vi "Lab Panel V5.24.2.vi"() -> ()   [LabVIEW 2013] (continued)
                          tunnel: w873 -> [_ w886]
                          tunnel: w872 -> [_ w885]
                          tunnel: [errorcluster {"status"=FALSE, "code"=0, "source"=""} ("error out") w884] -> w871
                          tunnel: w870 -> [_ w883]
                          tunnel: w869 -> [_ w882]
                          tunnel: w868 -> [_ w881]
                          tunnel: w867 -> [_ w880]
                          tunnel: w865 -> [_ w879]
                          frame False {
                            w877 = FALSE
                            n583 = local write "RUN LAB01-2"(w877) -> ()
                            n584 = local write "run lab01-2"(w877) -> ()
                          }
                          frame True {
                            n585 = stacked-sequence {
                              seq-local: [w890 _ _ _ _] -> [_ w914 _ _ _]
                              tunnel: w889 -> [w895 _ _ _ _]
                              tunnel: w888 -> [w892 _ _ _ _]
                              tunnel: w887 -> [w905 _ _ _ _]
                              tunnel: w886 -> [w898 _ _ _ _]
                              tunnel: w885 -> [w893 _ _ _ _]
                              tunnel: [_ w909 _ _ _] -> w884
                              tunnel: w883 -> [_ _ _ w936 _]
                              tunnel: w882 -> [_ _ _ w935 _]
                              tunnel: w881 -> [_ _ _ w934 _]
                              tunnel: w880 -> [_ _ _ _ _]
                              tunnel: w879 -> [_ _ _ _ w949]
                              frame #0 {
                                w891 = "\\"
                                n586 = local read "SET LAB01-2"() -> (w900:T5)
                                n587 = case shown="\"CYCLE TEST\"" w905 {
                                tunnel: ["L01-2-CHART TEST-" "L01-2-CYCLE TEST-" "L01-2-T-RISE TEST-"] -> w901
                                frame "CHART TEST", Default {
                                }
                                frame "CYCLE TEST" {
                                }
                                frame "T-RISE TEST" {
                                }
                                }
                                n588 = Unbundle(w900) -> ("DESCRIPTION"=w899:string)  [unwired: 4 out]
                                n589 = Concatenate Strings(w895, "\\", w893, w891, w892, w891) -> (w902:string)
                                n590 = String To Path(string=w902) -> (path=w904:path)
                                n591 = Concatenate Strings(w902, w901, w899, "-", w898, ".tdms") -> (w890:string)
                                n592 = Create Folder(path (use dialog)=w904) -> (error out=w903:errorcluster)  [unwired: 2 in, 2 out]
                                n593 = call <vilib>:"Clear Errors.vi"("error in (no error)"=w903) -> ()  [unwired: 6 in, 1 out]
                                n594 = global write "Global 1.vi" "LAB01-2 FILE"(w890) -> ()
                              }
                              frame #1 {
                                (unwired) FALSE
                                n595 = String To Path(string=w914) -> (path=w910:path)
                                n596 = TDMS Open(6:FALSE, 10:T21."create or replace" ("operation (0:open)"), 11:w910) -> (0:w909:errorcluster, 3:→"TDMS LAB01-2":refnum<k34>)  [unwired: 4 in]
                              }
                              frame #2 {
                                n597 = local read "SET LAB01-2"() -> (w920:T5)
                                n598 = local read "TDMS LAB01-2"() -> (w931:refnum<k34>)
                                n599 = Build Array("Testers Name", "Description", "Set Test Cycles", "T-Rise minutes", "T-Rise Deg C") -> (w921:string[])
                                n600 = Unbundle(w920) -> ("NAME"=w919:string, "DESCRIPTION"=w918:string, "CYCLES"=w917:dbl, "T-RISE mins"=w916:dbl, "T-RISE deg C"=w915:dbl)
                                n601 = Number To Decimal String(number=w917) -> (decimal integer string=w930:string)  [unwired: 1 in]
                                n602 = Number To Decimal String(number=w916) -> (decimal integer string=w929:string)  [unwired: 1 in]
                                n603 = Number To Decimal String(number=w915) -> (decimal integer string=w928:string)  [unwired: 1 in]
                                n604 = Build Array(w919, w918, w930, w929, w928) -> (w927:string[])
                                n605 = TDMS Set Properties(5:w927, 7:w921, 11:w931) -> ()  [unwired: 3 in, 4 out]
                              }
                              frame #3 {
                                n606 = local read "DISP LAB01-2"() -> (w933:T4)
                                n607 = Concatenate Strings("LAB01-2  ", w936) -> (w937:string)
                                n608 = Two Button Dialog(message=w937, 1:w934, 2:w935) -> (T button?=w939:bool)
                                n609 = case shown="True" w939 {
                                tunnel: w933 -> [w946 w947]
                                tunnel: [w946 w947] -> w943
                                tunnel: [w945 w948] -> w942
                                tunnel: [w944 w948] -> w941
                                frame False {
                                n610 = Unbundle(w946) -> ("CYCLE"=w945:dbl, "MINS"=w944:dbl)  [unwired: 1 out]
                                }
                                frame True {
                                w948 = 0.0
                                }
                                }
                                n611 = Bundle(cluster=w943, "CYCLE"=w942, "MINS"=w941, "STATUS"="RUN") -> (w932:T4)
                                n612 = local write "DISP LAB01-2"(w932) -> ()
                              }
                              frame #4 {
                                n613 = local read "TEMP START LAB01-2"() -> (w951:cluster{"TL":dbl, "TN":dbl})
                                n614 = Bundle(cluster=w951, "TL"=w949, "TN"=w949) -> (w950:cluster{"TL":dbl, "TN":dbl})
                                n615 = local write "TEMP START LAB01-2"(w950) -> ()
                              }
                            }
                          }
                        }
                      }
                    }
                  }
                }
              }
              event "RUN LAB02-1": Value Change {
                n616 = event-data() -> ("NewVal"=w957:bool)  [unwired: 1 in, 5 out]
                n617 = local read "SIG LAB02-1"() -> (w953:T2)
                n618 = case shown="True" w957 {
                  tunnel: w963 -> [_ w1001]
                  tunnel: w962 -> [_ w1000]
                  tunnel: w960 -> [w965 w999]
                  tunnel: w961 -> [_ w998]
                  tunnel: w959 -> [_ w997]
                  tunnel: [w964 w996] -> w958
                  tunnel: w956 -> [_ w995]
                  tunnel: w955 -> [_ w994]
                  tunnel: w954 -> [_ w993]
                  tunnel: w953 -> [_ w992]
                  tunnel: w952 -> [_ w991]
                  frame False {
                    # "stop test"
                    n619 = stacked-sequence {
                      tunnel: w965 -> [w974 _]
                      tunnel: [w966 _] -> w964
                      frame #0 {
                        n620 = local read "DISP LAB02-1"() -> (w973:T4)
                        n621 = Unbundle(w973) -> ("CYCLE"=w971:dbl, "MINS"=w972:dbl)  [unwired: 1 out]
                        n622 = case shown="\"CYCLE TEST\"" w974 {
                          tunnel: w972 -> [_ _ w981]
                          tunnel: w971 -> [w979 w980 _]
                          tunnel: [w979 w980 w981] -> w970
                          frame "CHART TEST", Default {
                          }
                          frame "CYCLE TEST" {
                          }
                          frame "T-RISE TEST" {
                          }
                        }
                        n623 = local read "TDMS LAB02-1"() -> (w978:refnum<k34>)
                        n624 = Build Array("STOPPED") -> (w975:string[])
                        n625 = Build Array(w970) -> (w969:dbl[])
                        n626 = TDMS Write(0:w978, 5:"TEST RESULT", 7:w975, 9:w969) -> (4:w967:refnum<k34>, 15:w968:errorcluster)  [unwired: 2 in, 2 out]
                        n627 = TDMS Close(8:w968, 11:w967) -> (0:w966:errorcluster)  [unwired: 1 out]
                      }
                      frame #1 {
                        n628 = local read "DISP LAB02-1"() -> (w985:T4)
                        n629 = stacked-sequence {
                          tunnel: "LAB02-1" -> [w987 w989]
                          frame #0 {
                            n630 = call "sub vi - defrag tdms v1.vi"("panel id"=w987) -> ("error out"=w986:errorcluster)  [unwired: 10 in]
                            n631 = local write "data file error"(w986) -> ()
                          }
                          frame #1 {
                            n632 = local write "RESULT LAB02-1"(FALSE) -> ()
                            n633 = call "Save data file (stop) v3.vi"("panel id"=w989) -> ("network file save error"=w988:errorcluster)  [unwired: 9 in, 1 out]
                            n634 = local write "data file error"(w988) -> ()
                          }
                        }
                        n635 = Bundle(cluster=w985, "STATUS"="STOP") -> (w983:T4)  [unwired: 2 in]
                        n636 = local write "DISP LAB02-1"(w983) -> ()
                      }
                    }
                  }
                  frame True {
                    n637 = stacked-sequence {
                      seq-local: [w1003 _] -> [_ w1007]
                      tunnel: w1001 -> [_ w1017]
                      tunnel: w1000 -> [_ w1016]
                      tunnel: w999 -> [_ w1015]
                      tunnel: w998 -> [_ w1014]
                      tunnel: w997 -> [_ w1013]
                      tunnel: [_ w1012] -> w996
                      tunnel: w995 -> [_ w1011]
                      tunnel: w994 -> [_ w1010]
                      tunnel: w993 -> [_ w1009]
                      tunnel: w992 -> [w1002 w1008]
                      tunnel: w991 -> [_ w1006]
                      frame #0 {
                        n638 = Unbundle(w1002) -> ("AMPS"=w1005:dbl)  [unwired: 4 out]
                        n639 = call "Check For Amps on v1.vi"("ID"="LAB02-1", "amps"=w1005) -> ("amps"=w1003:bool)  [unwired: 9 in]
                      }
                      frame #1 {
                        n640 = case shown="True" w1007 {
                          tunnel: w1017 -> [_ w1030]
                          tunnel: w1016 -> [_ w1029]
                          tunnel: w1015 -> [_ w1028]
                          tunnel: w1014 -> [_ w1027]
                          tunnel: w1013 -> [_ w1026]
                          tunnel: [errorcluster {"status"=FALSE, "code"=0, "source"=""} ("error out") w1025] -> w1012
                          tunnel: w1011 -> [_ w1024]
                          tunnel: w1010 -> [_ w1023]
                          tunnel: w1009 -> [_ w1022]
                          tunnel: w1008 -> [_ w1021]
                          tunnel: w1006 -> [_ w1020]
                          frame False {
                            w1019 = FALSE
                            n641 = local write "RUN LAB02-1"(w1019) -> ()
                            n642 = local write "run lab02-1"(w1019) -> ()
                          }
                          frame True {
                            n643 = stacked-sequence {
                              seq-local: [w1031 _ _ _ _] -> [_ w1055 _ _ _]
                              tunnel: w1030 -> [w1036 _ _ _ _]
                              tunnel: w1029 -> [w1033 _ _ _ _]
                              tunnel: w1028 -> [w1046 _ _ _ _]
                              tunnel: w1027 -> [w1039 _ _ _ _]
                              tunnel: w1026 -> [w1034 _ _ _ _]
                              tunnel: [_ w1050 _ _ _] -> w1025
                              tunnel: w1024 -> [_ _ _ w1076 _]
                              tunnel: w1023 -> [_ _ _ w1075 _]
                              tunnel: w1022 -> [_ _ _ w1074 _]
                              tunnel: w1021 -> [_ _ _ _ _]
                              tunnel: w1020 -> [_ _ _ _ w1090]
                              frame #0 {
                                w1032 = "\\"
                                n644 = local read "SET LAB02-1"() -> (w1041:T5)
                                n645 = case shown="\"CYCLE TEST\"" w1046 {
                                tunnel: ["L02-1-CHART TEST-" "L02-1-CYCLE TEST-" "L02-1-T-RISE TEST-"] -> w1042
                                frame "CHART TEST", Default {
                                }
                                frame "CYCLE TEST" {
                                }
                                frame "T-RISE TEST" {
                                }
                                }
                                n646 = Unbundle(w1041) -> ("DESCRIPTION"=w1040:string)  [unwired: 4 out]
                                n647 = Concatenate Strings(w1036, "\\", w1034, w1032, w1033, w1032) -> (w1043:string)
                                n648 = String To Path(string=w1043) -> (path=w1045:path)
                                n649 = Concatenate Strings(w1043, w1042, w1040, "-", w1039, ".tdms") -> (w1031:string)
                                n650 = Create Folder(path (use dialog)=w1045) -> (error out=w1044:errorcluster)  [unwired: 2 in, 2 out]
                                n651 = global write "Global 1.vi" "LAB02-1 FILE"(w1031) -> ()
                                n652 = call <vilib>:"Clear Errors.vi"("error in (no error)"=w1044) -> ()  [unwired: 6 in, 1 out]
                              }
                              frame #1 {
                                (unwired) FALSE
                                n653 = String To Path(string=w1055) -> (path=w1051:path)
                                n654 = TDMS Open(6:FALSE, 10:T21."create or replace" ("operation (0:open)"), 11:w1051) -> (0:w1050:errorcluster, 3:→"TDMS LAB02-1":refnum<k34>)  [unwired: 4 in]
                              }
                              frame #2 {
                                n655 = local read "SET LAB02-1"() -> (w1061:T5)
                                n656 = local read "TDMS LAB02-1"() -> (w1072:refnum<k34>)
                                n657 = Build Array("Testers Name", "Description", "Set Test Cycles", "T-Rise minutes", "T-Rise Deg C") -> (w1062:string[])
                                n658 = Unbundle(w1061) -> ("NAME"=w1060:string, "DESCRIPTION"=w1059:string, "CYCLES"=w1058:dbl, "T-RISE mins"=w1057:dbl, "T-RISE deg C"=w1056:dbl)
                                n659 = Number To Decimal String(number=w1058) -> (decimal integer string=w1071:string)  [unwired: 1 in]
                                n660 = Number To Decimal String(number=w1057) -> (decimal integer string=w1070:string)  [unwired: 1 in]
                                n661 = Number To Decimal String(number=w1056) -> (decimal integer string=w1069:string)  [unwired: 1 in]
                                n662 = Build Array(w1060, w1059, w1071, w1070, w1069) -> (w1068:string[])
                                n663 = TDMS Set Properties(5:w1068, 7:w1062, 11:w1072) -> ()  [unwired: 3 in, 4 out]
                              }
                              frame #3 {
                                n664 = local read "DISP LAB02-1"() -> (w1077:T4)
                                n665 = Concatenate Strings("LAB02-1  ", w1076) -> (w1078:string)
                                n666 = Two Button Dialog(message=w1078, 1:w1074, 2:w1075) -> (T button?=w1080:bool)
                                n667 = case shown="True" w1080 {
                                tunnel: w1077 -> [w1087 w1088]
                                tunnel: [w1087 w1088] -> w1084
                                tunnel: [w1086 w1089] -> w1083
                                tunnel: [w1085 w1089] -> w1082
                                frame False {
                                n668 = Unbundle(w1087) -> ("CYCLE"=w1086:dbl, "MINS"=w1085:dbl)  [unwired: 1 out]
                                }
                                frame True {
                                w1089 = 0.0
                                }
                                }
                                n669 = Bundle(cluster=w1084, "CYCLE"=w1083, "MINS"=w1082, "STATUS"="RUN") -> (w1073:T4)
                                n670 = local write "DISP LAB02-1"(w1073) -> ()
                              }
                              frame #4 {
                                n671 = local read "TEMP START LAB02-1"() -> (w1092:cluster{"TL":dbl, "TN":dbl})
                                n672 = Bundle(cluster=w1092, "TL"=w1090, "TN"=w1090) -> (w1091:cluster{"TL":dbl, "TN":dbl})
                                n673 = local write "TEMP START LAB02-1"(w1091) -> ()
                              }
                            }
                          }
                        }
                      }
                    }
                  }
                }
                n674 = local write "run lab02-1"(w957) -> ()
              }
              event "RUN LAB02-2": Value Change {
                n675 = event-data() -> ("NewVal"=w1097:bool)  [unwired: 1 in, 5 out]
                n676 = local write "run lab02-2"(w1097) -> ()
                n677 = case shown="True" w1097 {
                  tunnel: w1103 -> [_ w1141]
                  tunnel: w1102 -> [_ w1140]
                  tunnel: w1100 -> [w1105 w1139]
                  tunnel: w1101 -> [_ w1138]
                  tunnel: w1099 -> [_ w1137]
                  tunnel: [w1104 w1136] -> w1098
                  tunnel: w1096 -> [_ w1135]
                  tunnel: w1095 -> [_ w1134]
                  tunnel: w1094 -> [_ w1133]
                  tunnel: w1093 -> [_ w1131]
                  frame False {
                    # "stop test"
                    n678 = stacked-sequence {
                      tunnel: w1105 -> [w1114 _]
                      tunnel: [w1106 _] -> w1104
                      frame #0 {
                        n679 = local read "DISP LAB02-2"() -> (w1113:T4)
                        n680 = Unbundle(w1113) -> ("CYCLE"=w1111:dbl, "MINS"=w1112:dbl)  [unwired: 1 out]
                        n681 = case shown="\"CYCLE TEST\"" w1114 {
                          tunnel: w1112 -> [_ _ w1121]
                          tunnel: w1111 -> [w1119 w1120 _]
                          tunnel: [w1119 w1120 w1121] -> w1110
                          frame "CHART TEST", Default {
                          }
                          frame "CYCLE TEST" {
                          }
                          frame "T-RISE TEST" {
                          }
                        }
                        n682 = local read "TDMS LAB02-2"() -> (w1118:refnum<k34>)
                        n683 = Build Array("STOPPED") -> (w1115:string[])
                        n684 = Build Array(w1110) -> (w1109:dbl[])
                        n685 = TDMS Write(0:w1118, 5:"TEST RESULT", 7:w1115, 9:w1109) -> (4:w1107:refnum<k34>, 15:w1108:errorcluster)  [unwired: 2 in, 2 out]
                        n686 = TDMS Close(8:w1108, 11:w1107) -> (0:w1106:errorcluster)  [unwired: 1 out]
                      }
                      frame #1 {
                        n687 = local read "DISP LAB02-2"() -> (w1125:T4)
                        n688 = stacked-sequence {
                          tunnel: "LAB02-2" -> [w1127 w1129]
                          frame #0 {
                            n689 = call "sub vi - defrag tdms v1.vi"("panel id"=w1127) -> ("error out"=w1126:errorcluster)  [unwired: 10 in]
                            n690 = local write "data file error"(w1126) -> ()
                          }
                          frame #1 {
                            n691 = call "Save data file (stop) v3.vi"("panel id"=w1129) -> ("network file save error"=w1128:errorcluster)  [unwired: 9 in, 1 out]
                            n692 = local write "RESULT LAB02-2"(FALSE) -> ()
                            n693 = local write "data file error"(w1128) -> ()
                          }
                        }
                        n694 = Bundle(cluster=w1125, "STATUS"="STOP") -> (w1123:T4)  [unwired: 2 in]
                        n695 = local write "DISP LAB02-2"(w1123) -> ()
                      }
                    }
                  }
                  frame True {
                    n696 = local read "SIG LAB02-2"() -> (w1132:T2)
                    n697 = stacked-sequence {
                      seq-local: [w1143 _] -> [_ w1147]
                      tunnel: w1141 -> [_ w1157]
                      tunnel: w1140 -> [_ w1156]
                      tunnel: w1139 -> [_ w1155]
                      tunnel: w1138 -> [_ w1154]
                      tunnel: w1137 -> [_ w1153]
                      tunnel: [_ w1152] -> w1136
                      tunnel: w1135 -> [_ w1151]
                      tunnel: w1134 -> [_ w1150]
                      tunnel: w1133 -> [_ w1149]
                      tunnel: w1132 -> [w1142 w1148]
                      tunnel: w1131 -> [_ w1146]
                      frame #0 {
                        n698 = Unbundle(w1142) -> ("AMPS"=w1145:dbl)  [unwired: 4 out]
                        n699 = call "Check For Amps on v1.vi"("ID"="LAB02-2", "amps"=w1145) -> ("amps"=w1143:bool)  [unwired: 9 in]
                      }
                      frame #1 {
                        n700 = case shown="True" w1147 {
                          tunnel: w1157 -> [_ w1170]
                          tunnel: w1156 -> [_ w1169]
                          tunnel: w1155 -> [_ w1168]
                          tunnel: w1154 -> [_ w1167]
                          tunnel: w1153 -> [_ w1166]
                          tunnel: [errorcluster {"status"=FALSE, "code"=0, "source"=""} ("error out") w1165] -> w1152
                          tunnel: w1151 -> [_ w1164]
                          tunnel: w1150 -> [_ w1163]
                          tunnel: w1149 -> [_ w1162]
                          tunnel: w1148 -> [_ w1161]
                          tunnel: w1146 -> [_ w1160]
                          frame False {
                            w1158 = FALSE
                            n701 = local write "RUN LAB02-2"(w1158) -> ()
                            n702 = local write "run lab02-2"(w1158) -> ()
                          }
                          frame True {
                            n703 = stacked-sequence {
                              seq-local: [w1171 _ _ _ _] -> [_ w1195 _ _ _]
                              tunnel: w1170 -> [w1176 _ _ _ _]
                              tunnel: w1169 -> [w1173 _ _ _ _]
                              tunnel: w1168 -> [w1186 _ _ _ _]
                              tunnel: w1167 -> [w1179 _ _ _ _]
                              tunnel: w1166 -> [w1174 _ _ _ _]
                              tunnel: [_ w1190 _ _ _] -> w1165
                              tunnel: w1164 -> [_ _ _ w1216 _]
                              tunnel: w1163 -> [_ _ _ w1215 _]
                              tunnel: w1162 -> [_ _ _ w1214 _]
                              tunnel: w1161 -> [_ _ _ _ _]
                              tunnel: w1160 -> [_ _ _ _ w1230]
                              frame #0 {
                                w1172 = "\\"
                                n704 = local read "SET LAB02-2"() -> (w1181:T5)
                                n705 = case shown="\"CYCLE TEST\"" w1186 {
                                tunnel: ["L02-2-CHART TEST-" "L02-2-CYCLE TEST-" "L02-2-T-RISE TEST-"] -> w1182
                                frame "CHART TEST", Default {
                                }
                                frame "CYCLE TEST" {
                                }
                                frame "T-RISE TEST" {
                                }
                                }
                                n706 = Unbundle(w1181) -> ("DESCRIPTION"=w1180:string)  [unwired: 4 out]
                                n707 = Concatenate Strings(w1176, "\\", w1174, w1172, w1173, w1172) -> (w1183:string)
                                n708 = String To Path(string=w1183) -> (path=w1185:path)
                                n709 = Concatenate Strings(w1183, w1182, w1180, "-", w1179, ".tdms") -> (w1171:string)
                                n710 = Create Folder(path (use dialog)=w1185) -> (error out=w1184:errorcluster)  [unwired: 2 in, 2 out]
                                n711 = global write "Global 1.vi" "LAB02-2 FILE"(w1171) -> ()
                                n712 = call <vilib>:"Clear Errors.vi"("error in (no error)"=w1184) -> ()  [unwired: 6 in, 1 out]
                              }
                              frame #1 {
                                (unwired) FALSE
                                n713 = String To Path(string=w1195) -> (path=w1191:path)
                                n714 = TDMS Open(6:FALSE, 10:T21."create or replace" ("operation (0:open)"), 11:w1191) -> (0:w1190:errorcluster, 3:→"TDMS LAB02-2":refnum<k34>)  [unwired: 4 in]
                              }
                              frame #2 {
                                n715 = local read "SET LAB02-2"() -> (w1201:T5)
                                n716 = local read "TDMS LAB02-2"() -> (w1212:refnum<k34>)
                                n717 = Build Array("Testers Name", "Description", "Set Test Cycles", "T-Rise minutes", "T-Rise Deg C") -> (w1202:string[])
                                n718 = Unbundle(w1201) -> ("NAME"=w1200:string, "DESCRIPTION"=w1199:string, "CYCLES"=w1198:dbl, "T-RISE mins"=w1197:dbl, "T-RISE deg C"=w1196:dbl)
                                n719 = Number To Decimal String(number=w1198) -> (decimal integer string=w1211:string)  [unwired: 1 in]
                                n720 = Number To Decimal String(number=w1197) -> (decimal integer string=w1210:string)  [unwired: 1 in]
                                n721 = Number To Decimal String(number=w1196) -> (decimal integer string=w1209:string)  [unwired: 1 in]
                                n722 = Build Array(w1200, w1199, w1211, w1210, w1209) -> (w1208:string[])
                                n723 = TDMS Set Properties(5:w1208, 7:w1202, 11:w1212) -> ()  [unwired: 3 in, 4 out]
                              }
                              frame #3 {
                                n724 = local read "DISP LAB02-2"() -> (w1217:T4)
                                n725 = Concatenate Strings("LAB02-2  ", w1216) -> (w1218:string)
                                n726 = Two Button Dialog(message=w1218, 1:w1214, 2:w1215) -> (T button?=w1220:bool)
                                n727 = case shown="True" w1220 {
                                tunnel: w1217 -> [w1227 w1228]
                                tunnel: [w1227 w1228] -> w1224
                                tunnel: [w1226 w1229] -> w1223
                                tunnel: [w1225 w1229] -> w1222
                                frame False {
                                n728 = Unbundle(w1227) -> ("CYCLE"=w1226:dbl, "MINS"=w1225:dbl)  [unwired: 1 out]
                                }
                                frame True {
                                w1229 = 0.0
                                }
                                }
                                n729 = Bundle(cluster=w1224, "CYCLE"=w1223, "MINS"=w1222, "STATUS"="RUN") -> (w1213:T4)
                                n730 = local write "DISP LAB02-2"(w1213) -> ()
                              }
                              frame #4 {
                                n731 = local read "TEMP START LAB02-2"() -> (w1232:cluster{"TL":dbl, "TN":dbl})
                                n732 = Bundle(cluster=w1232, "TL"=w1230, "TN"=w1230) -> (w1231:cluster{"TL":dbl, "TN":dbl})
                                n733 = local write "TEMP START LAB02-2"(w1231) -> ()
                              }
                            }
                          }
                        }
                      }
                    }
                  }
                }
              }
              event "RUN LAB03-1": Value Change {
                n734 = event-data() -> ("NewVal"=w1237:bool)  [unwired: 1 in, 5 out]
                n735 = local write "run lab03-1"(w1237) -> ()
                n736 = case shown="True" w1237 {
                  tunnel: w1243 -> [_ w1281]
                  tunnel: w1242 -> [_ w1280]
                  tunnel: w1240 -> [w1245 w1279]
                  tunnel: w1241 -> [_ w1278]
                  tunnel: w1239 -> [_ w1277]
                  tunnel: [w1244 w1276] -> w1238
                  tunnel: w1236 -> [_ w1275]
                  tunnel: w1235 -> [_ w1274]
                  tunnel: w1234 -> [_ w1273]
                  tunnel: w1233 -> [_ w1271]
                  frame False {
                    # "stop test"
                    n737 = stacked-sequence {
                      tunnel: w1245 -> [w1254 _]
                      tunnel: [w1246 _] -> w1244
                      frame #0 {
                        n738 = local read "DISP LAB03-1"() -> (w1253:T4)
                        n739 = Unbundle(w1253) -> ("CYCLE"=w1251:dbl, "MINS"=w1252:dbl)  [unwired: 1 out]
                        n740 = case shown="\"CYCLE TEST\"" w1254 {
                          tunnel: w1252 -> [_ _ w1261]
                          tunnel: w1251 -> [w1259 w1260 _]
                          tunnel: [w1259 w1260 w1261] -> w1250
                          frame "CHART TEST", Default {
                          }
                          frame "CYCLE TEST" {
                          }
                          frame "T-RISE TEST" {
                          }
                        }
                        n741 = local read "TDMS LAB03-1"() -> (w1258:refnum<k34>)
                        n742 = Build Array("STOPPED") -> (w1255:string[])
                        n743 = Build Array(w1250) -> (w1249:dbl[])
                        n744 = TDMS Write(0:w1258, 5:"TEST RESULT", 7:w1255, 9:w1249) -> (4:w1247:refnum<k34>, 15:w1248:errorcluster)  [unwired: 2 in, 2 out]
                        n745 = TDMS Close(8:w1248, 11:w1247) -> (0:w1246:errorcluster)  [unwired: 1 out]
                      }
                      frame #1 {
                        n746 = local read "DISP LAB03-1"() -> (w1265:T4)
                        n747 = stacked-sequence {
                          tunnel: "LAB03-1" -> [w1267 w1269]
                          frame #0 {
                            n748 = call "sub vi - defrag tdms v1.vi"("panel id"=w1267) -> ("error out"=w1266:errorcluster)  [unwired: 10 in]
                            n749 = local write "data file error"(w1266) -> ()
                          }
                          frame #1 {
                            n750 = call "Save data file (stop) v3.vi"("panel id"=w1269) -> ("network file save error"=w1268:errorcluster)  [unwired: 9 in, 1 out]
                            n751 = local write "RESULT LAB03-1"(FALSE) -> ()
                            n752 = local write "data file error"(w1268) -> ()
                          }
                        }
                        n753 = Bundle(cluster=w1265, "STATUS"="STOP") -> (w1263:T4)  [unwired: 2 in]
                        n754 = local write "DISP LAB03-1"(w1263) -> ()
                      }
                    }
                  }
                  frame True {
                    n755 = local read "SIG LAB03-1"() -> (w1272:T2)
                    n756 = stacked-sequence {
                      seq-local: [w1283 _] -> [_ w1287]
                      tunnel: w1281 -> [_ w1297]
                      tunnel: w1280 -> [_ w1296]
                      tunnel: w1279 -> [_ w1295]
                      tunnel: w1278 -> [_ w1294]
                      tunnel: w1277 -> [_ w1293]
                      tunnel: [_ w1292] -> w1276
                      tunnel: w1275 -> [_ w1291]
                      tunnel: w1274 -> [_ w1290]
                      tunnel: w1273 -> [_ w1289]
                      tunnel: w1272 -> [w1282 w1288]
                      tunnel: w1271 -> [_ w1286]
                      frame #0 {
                        n757 = Unbundle(w1282) -> ("AMPS"=w1285:dbl)  [unwired: 4 out]
                        n758 = call "Check For Amps on v1.vi"("ID"="LAB03-1", "amps"=w1285) -> ("amps"=w1283:bool)  [unwired: 9 in]
                      }
                      frame #1 {
                        n759 = case shown="True" w1287 {
                          tunnel: w1297 -> [_ w1310]
                          tunnel: w1296 -> [_ w1309]
                          tunnel: w1295 -> [_ w1308]
                          tunnel: w1294 -> [_ w1307]
                          tunnel: w1293 -> [_ w1306]
                          tunnel: [errorcluster {"status"=FALSE, "code"=0, "source"=""} ("error out") w1305] -> w1292
                          tunnel: w1291 -> [_ w1304]
                          tunnel: w1290 -> [_ w1303]
                          tunnel: w1289 -> [_ w1302]
                          tunnel: w1288 -> [_ w1301]
                          tunnel: w1286 -> [_ w1300]
                          frame False {
                            w1298 = FALSE
                            n760 = local write "RUN LAB03-1"(w1298) -> ()
                            n761 = local write "run lab03-1"(w1298) -> ()
                          }
                          frame True {
                            n762 = stacked-sequence {
                              seq-local: [w1311 _ _ _ _] -> [_ w1335 _ _ _]
                              tunnel: w1310 -> [w1316 _ _ _ _]
                              tunnel: w1309 -> [w1313 _ _ _ _]
                              tunnel: w1308 -> [w1326 _ _ _ _]
                              tunnel: w1307 -> [w1319 _ _ _ _]
                              tunnel: w1306 -> [w1314 _ _ _ _]
                              tunnel: [_ w1330 _ _ _] -> w1305
                              tunnel: w1304 -> [_ _ _ w1355 _]
                              tunnel: w1303 -> [_ _ _ w1354 _]
                              tunnel: w1302 -> [_ _ _ w1353 _]
                              tunnel: w1301 -> [_ _ _ _ _]
                              tunnel: w1300 -> [_ _ _ _ w1370]
                              frame #0 {
                                w1312 = "\\"
                                n763 = local read "SET LAB03-1"() -> (w1321:T5)
                                n764 = case shown="\"T-RISE TEST\"" w1326 {
                                tunnel: ["L03-1-CHART TEST-" "L03-1-CYCLE TEST-" "L03-1-T-RISE TEST-"] -> w1322
                                frame "CHART TEST", Default {
                                }
                                frame "CYCLE TEST" {
                                }
                                frame "T-RISE TEST" {
                                }
                                }
                                n765 = Unbundle(w1321) -> ("DESCRIPTION"=w1320:string)  [unwired: 4 out]
                                n766 = Concatenate Strings(w1316, "\\", w1314, w1312, w1313, w1312) -> (w1323:string)
                                n767 = String To Path(string=w1323) -> (path=w1325:path)
                                n768 = Concatenate Strings(w1323, w1322, w1320, "-", w1319, ".tdms") -> (w1311:string)
                                n769 = Create Folder(path (use dialog)=w1325) -> (error out=w1324:errorcluster)  [unwired: 2 in, 2 out]
                                n770 = global write "Global 1.vi" "LAB03-1 FILE"(w1311) -> ()
                                n771 = call <vilib>:"Clear Errors.vi"("error in (no error)"=w1324) -> ()  [unwired: 6 in, 1 out]
                              }
                              frame #1 {
                                (unwired) FALSE
                                n772 = String To Path(string=w1335) -> (path=w1331:path)
                                n773 = TDMS Open(6:FALSE, 10:T21."create or replace" ("operation (0:open)"), 11:w1331) -> (0:w1330:errorcluster, 3:→"TDMS LAB03-1":refnum<k34>)  [unwired: 4 in]
                              }
                              frame #2 {
                                n774 = local read "SET LAB03-1"() -> (w1341:T5)
                                n775 = local read "TDMS LAB03-1"() -> (w1352:refnum<k34>)
                                n776 = Build Array("Testers Name", "Description", "Set Test Cycles", "T-Rise minutes", "T-Rise Deg C") -> (w1342:string[])
                                n777 = Unbundle(w1341) -> ("NAME"=w1340:string, "DESCRIPTION"=w1339:string, "CYCLES"=w1338:dbl, "T-RISE mins"=w1337:dbl, "T-RISE deg C"=w1336:dbl)
                                n778 = Number To Decimal String(number=w1338) -> (decimal integer string=w1351:string)  [unwired: 1 in]
                                n779 = Number To Decimal String(number=w1337) -> (decimal integer string=w1350:string)  [unwired: 1 in]
                                n780 = Number To Decimal String(number=w1336) -> (decimal integer string=w1349:string)  [unwired: 1 in]
                                n781 = Build Array(w1340, w1339, w1351, w1350, w1349) -> (w1348:string[])
                                n782 = TDMS Set Properties(5:w1348, 7:w1342, 11:w1352) -> ()  [unwired: 3 in, 4 out]
                              }
                              frame #3 {
                                n783 = local read "DISP LAB03-1"() -> (w1357:T4)
                                n784 = Concatenate Strings("LAB03-1  ", w1355) -> (w1358:string)
                                n785 = Two Button Dialog(message=w1358, 1:w1353, 2:w1354) -> (T button?=w1360:bool)
                                n786 = case shown="True" w1360 {
                                tunnel: w1357 -> [w1367 w1368]
                                tunnel: [w1367 w1368] -> w1364
                                tunnel: [w1366 w1369] -> w1363
                                tunnel: [w1365 w1369] -> w1362
                                frame False {
                                n787 = Unbundle(w1367) -> ("CYCLE"=w1366:dbl, "MINS"=w1365:dbl)  [unwired: 1 out]
                                }
                                frame True {
                                w1369 = 0.0
                                }
                                }
                                n788 = Bundle(cluster=w1364, "CYCLE"=w1363, "MINS"=w1362, "STATUS"="RUN") -> (w1356:T4)
                                n789 = local write "DISP LAB03-1"(w1356) -> ()
                              }
                              frame #4 {
                                n790 = local read "TEMP START LAB03-1"() -> (w1372:cluster{"TL":dbl, "TN":dbl})
                                n791 = Bundle(cluster=w1372, "TL"=w1370, "TN"=w1370) -> (w1371:cluster{"TL":dbl, "TN":dbl})
                                n792 = local write "TEMP START LAB03-1"(w1371) -> ()
                              }
                            }
                          }
                        }
                      }
                    }
                  }
                }
              }
              event "RUN LAB03-2": Value Change {
                n793 = event-data() -> ("NewVal"=w1377:bool)  [unwired: 1 in, 5 out]
                n794 = local write "run lab03-2"(w1377) -> ()
                n795 = case shown="True" w1377 {
                  tunnel: w1383 -> [_ w1421]
                  tunnel: w1382 -> [_ w1420]
                  tunnel: w1380 -> [w1385 w1419]
                  tunnel: w1381 -> [_ w1418]
                  tunnel: w1379 -> [_ w1417]
                  tunnel: [w1384 w1416] -> w1378
                  tunnel: w1376 -> [_ w1415]
                  tunnel: w1375 -> [_ w1414]
                  tunnel: w1374 -> [_ w1413]
                  tunnel: w1373 -> [_ w1411]
                  frame False {
                    # "stop test"
                    n796 = stacked-sequence {
                      tunnel: w1385 -> [w1394 _]
                      tunnel: [w1386 _] -> w1384
                      frame #0 {
                        n797 = local read "DISP LAB03-2"() -> (w1393:T4)
                        n798 = Unbundle(w1393) -> ("CYCLE"=w1391:dbl, "MINS"=w1392:dbl)  [unwired: 1 out]
                        n799 = case shown="\"CYCLE TEST\"" w1394 {
                          tunnel: w1392 -> [_ _ w1401]
                          tunnel: w1391 -> [w1399 w1400 _]
                          tunnel: [w1399 w1400 w1401] -> w1390
                          frame "CHART TEST", Default {
                          }
                          frame "CYCLE TEST" {
                          }
                          frame "T-RISE TEST" {
                          }
                        }
                        n800 = local read "TDMS LAB03-2"() -> (w1398:refnum<k34>)
                        n801 = Build Array("STOPPED") -> (w1395:string[])
                        n802 = Build Array(w1390) -> (w1389:dbl[])
                        n803 = TDMS Write(0:w1398, 5:"TEST RESULT", 7:w1395, 9:w1389) -> (4:w1387:refnum<k34>, 15:w1388:errorcluster)  [unwired: 2 in, 2 out]
                        n804 = TDMS Close(8:w1388, 11:w1387) -> (0:w1386:errorcluster)  [unwired: 1 out]
                      }
                      frame #1 {
                        n805 = local read "DISP LAB03-2"() -> (w1405:T4)
                        n806 = stacked-sequence {
                          tunnel: "LAB03-2" -> [w1407 w1409]
                          frame #0 {
                            n807 = call "sub vi - defrag tdms v1.vi"("panel id"=w1407) -> ("error out"=w1406:errorcluster)  [unwired: 10 in]
                            n808 = local write "data file error"(w1406) -> ()
                          }
                          frame #1 {
                            n809 = call "Save data file (stop) v3.vi"("panel id"=w1409) -> ("network file save error"=w1408:errorcluster)  [unwired: 9 in, 1 out]
                            n810 = local write "RESULT LAB03-2"(FALSE) -> ()
                            n811 = local write "data file error"(w1408) -> ()
                          }
                        }
                        n812 = Bundle(cluster=w1405, "STATUS"="STOP") -> (w1403:T4)  [unwired: 2 in]
                        n813 = local write "DISP LAB03-2"(w1403) -> ()
                      }
                    }
                  }
                  frame True {
                    n814 = local read "SIG LAB03-2"() -> (w1412:T2)
                    n815 = stacked-sequence {
                      seq-local: [w1423 _] -> [_ w1427]
                      tunnel: w1421 -> [_ w1437]
                      tunnel: w1420 -> [_ w1436]
                      tunnel: w1419 -> [_ w1435]
                      tunnel: w1418 -> [_ w1434]
                      tunnel: w1417 -> [_ w1433]
                      tunnel: [_ w1432] -> w1416
                      tunnel: w1415 -> [_ w1431]
                      tunnel: w1414 -> [_ w1430]
                      tunnel: w1413 -> [_ w1429]
                      tunnel: w1412 -> [w1422 w1428]
                      tunnel: w1411 -> [_ w1426]
                      frame #0 {
                        n816 = Unbundle(w1422) -> ("AMPS"=w1425:dbl)  [unwired: 4 out]
                        n817 = call "Check For Amps on v1.vi"("ID"="LAB03-2", "amps"=w1425) -> ("amps"=w1423:bool)  [unwired: 9 in]
                      }
                      frame #1 {
                        n818 = case shown="True" w1427 {
                          tunnel: w1437 -> [_ w1450]
                          tunnel: w1436 -> [_ w1449]
                          tunnel: w1435 -> [_ w1448]
                          tunnel: w1434 -> [_ w1447]
                          tunnel: w1433 -> [_ w1446]
                          tunnel: [errorcluster {"status"=FALSE, "code"=0, "source"=""} ("error out") w1445] -> w1432
                          tunnel: w1431 -> [_ w1444]
                          tunnel: w1430 -> [_ w1443]
                          tunnel: w1429 -> [_ w1442]
                          tunnel: w1428 -> [_ w1441]
                          tunnel: w1426 -> [_ w1440]
                          frame False {
                            w1438 = FALSE
                            n819 = local write "RUN LAB03-2"(w1438) -> ()
                            n820 = local write "run lab03-2"(w1438) -> ()
                          }
                          frame True {
                            n821 = stacked-sequence {
                              seq-local: [w1451 _ _ _ _] -> [_ w1475 _ _ _]
                              tunnel: w1450 -> [w1456 _ _ _ _]
                              tunnel: w1449 -> [w1453 _ _ _ _]
                              tunnel: w1448 -> [w1466 _ _ _ _]
                              tunnel: w1447 -> [w1459 _ _ _ _]
                              tunnel: w1446 -> [w1454 _ _ _ _]
                              tunnel: [_ w1470 _ _ _] -> w1445
                              tunnel: w1444 -> [_ _ _ w1496 _]
                              tunnel: w1443 -> [_ _ _ w1495 _]
                              tunnel: w1442 -> [_ _ _ w1494 _]
                              tunnel: w1441 -> [_ _ _ _ _]
                              tunnel: w1440 -> [_ _ _ _ w1510]
                              frame #0 {
                                w1452 = "\\"
                                n822 = local read "SET LAB03-2"() -> (w1461:T5)
                                n823 = case shown="\"T-RISE TEST\"" w1466 {
                                tunnel: ["L03-2-CHART TEST-" "L03-2-CYCLE TEST-" "L03-2-T-RISE TEST-"] -> w1462
                                frame "CHART TEST", Default {
                                }
                                frame "CYCLE TEST" {
                                }
                                frame "T-RISE TEST" {
                                }
                                }
                                n824 = Unbundle(w1461) -> ("DESCRIPTION"=w1460:string)  [unwired: 4 out]
                                n825 = Concatenate Strings(w1456, "\\", w1454, w1452, w1453, w1452) -> (w1463:string)
                                n826 = String To Path(string=w1463) -> (path=w1465:path)
                                n827 = Concatenate Strings(w1463, w1462, w1460, "-", w1459, ".tdms") -> (w1451:string)
                                n828 = Create Folder(path (use dialog)=w1465) -> (error out=w1464:errorcluster)  [unwired: 2 in, 2 out]
                                n829 = global write "Global 1.vi" "LAB03-2 FILE"(w1451) -> ()
                                n830 = call <vilib>:"Clear Errors.vi"("error in (no error)"=w1464) -> ()  [unwired: 6 in, 1 out]
                              }
                              frame #1 {
                                (unwired) FALSE
                                n831 = String To Path(string=w1475) -> (path=w1471:path)
                                n832 = TDMS Open(6:FALSE, 10:T21."create or replace" ("operation (0:open)"), 11:w1471) -> (0:w1470:errorcluster, 3:→"TDMS LAB03-2":refnum<k34>)  [unwired: 4 in]
                              }
                              frame #2 {
                                n833 = local read "SET LAB03-2"() -> (w1481:T5)
                                n834 = local read "TDMS LAB03-2"() -> (w1492:refnum<k34>)
                                n835 = Build Array("Testers Name", "Description", "Set Test Cycles", "T-Rise minutes", "T-Rise Deg C") -> (w1482:string[])
                                n836 = Unbundle(w1481) -> ("NAME"=w1480:string, "DESCRIPTION"=w1479:string, "CYCLES"=w1478:dbl, "T-RISE mins"=w1477:dbl, "T-RISE deg C"=w1476:dbl)
                                n837 = Number To Decimal String(number=w1478) -> (decimal integer string=w1491:string)  [unwired: 1 in]
                                n838 = Number To Decimal String(number=w1477) -> (decimal integer string=w1490:string)  [unwired: 1 in]
                                n839 = Number To Decimal String(number=w1476) -> (decimal integer string=w1489:string)  [unwired: 1 in]
                                n840 = Build Array(w1480, w1479, w1491, w1490, w1489) -> (w1488:string[])
                                n841 = TDMS Set Properties(5:w1488, 7:w1482, 11:w1492) -> ()  [unwired: 3 in, 4 out]
                              }
                              frame #3 {
                                n842 = local read "DISP LAB03-2"() -> (w1497:T4)
                                n843 = Concatenate Strings("LAB03-2  ", w1496) -> (w1498:string)
                                n844 = Two Button Dialog(message=w1498, 1:w1494, 2:w1495) -> (T button?=w1500:bool)
                                n845 = case shown="True" w1500 {
                                tunnel: w1497 -> [w1507 w1508]
                                tunnel: [w1507 w1508] -> w1504
                                tunnel: [w1506 w1509] -> w1503
                                tunnel: [w1505 w1509] -> w1502
                                frame False {
                                n846 = Unbundle(w1507) -> ("CYCLE"=w1506:dbl, "MINS"=w1505:dbl)  [unwired: 1 out]
                                }
                                frame True {
                                w1509 = 0.0
                                }
                                }
                                n847 = Bundle(cluster=w1504, "CYCLE"=w1503, "MINS"=w1502, "STATUS"="RUN") -> (w1493:T4)
                                n848 = local write "DISP LAB03-2"(w1493) -> ()
                              }
                              frame #4 {
                                n849 = local read "TEMP START LAB03-2"() -> (w1512:cluster{"TL":dbl, "TN":dbl})
                                n850 = Bundle(cluster=w1512, "TL"=w1510, "TN"=w1510) -> (w1511:cluster{"TL":dbl, "TN":dbl})
                                n851 = local write "TEMP START LAB03-2"(w1511) -> ()
                              }
                            }
                          }
                        }
                      }
                    }
                  }
                }
              }
              event "RUN LAB04-1": Value Change {
